vi "LIA 48Bits Slicer.vi"(11 "m_axis_dout_tdata":fxp<+,48,48>) -> (2 "Y":fxp<+/-,22,2> format="%.21g", 3 "X":fxp<+/-,22,2> format="%.21g")   [LabVIEW 2017]
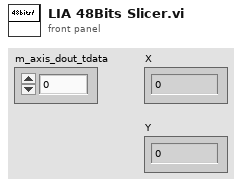
[diagram p1: front panel]
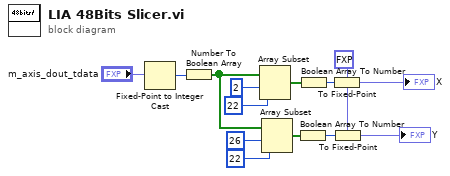
[diagram p0: block diagram]
diagram:
  w11 = fxp<+/-,22,2> 0.0 ("fixed-point type")
  n1 = Fixed-Point to Integer Cast(1:"m_axis_dout_tdata") -> (0:w1:u64)
  n2 = Number To Boolean Array(number=w1) -> (Boolean array=w2:bool[])
  n3 = Array Subset(array=w2, index=2, length=22) -> (w7:bool[])
  n4 = Array Subset(array=w2, index=26, length=22) -> (w8:bool[])
  n5 = Boolean Array To Number(Boolean array=w8) -> (number=w10:u32)
  n6 = Boolean Array To Number(Boolean array=w7) -> (number=w9:u32)
  n7 = To Fixed-Point(fixed-point type=w11, number=w9) -> (fixed-point=→"X":fxp<+/-,22,2>)
  n8 = To Fixed-Point(fixed-point type=w11, number=w10) -> (fixed-point=→"Y":fxp<+/-,22,2>)
